vi "AutoLin Protokoll Soll-Ist Abweichung.vi"(10 "Istwerte (ppm)":sgl[](array[numeric]), 11 "Sollwerte (ppm)":sgl[](array[numeric])) -> (1 "% vom Endwert":sgl[](array[numeric]), 2 "% vom Sollwert":sgl[](array[numeric]), 3 "abs. Fehler (ppm)":sgl[](array[numeric]))   [LabVIEW 2020, in "Linearisierung v2.lvlib" / "AutoLin Protokoll.lvlib"]
doc: "Berechnet bei der Kalibrierung die Abweichung der Messdaten des Messgerätes von den Kalibriervorgaben des Gasteilers.\n\nEingangsdaten: 1D-Arrays (SGL) mit N Konzentrationswerten in ppm\n Sollwerte (ppm): Konzentrationswerte Gasteiler\n Istwerte (ppm): Konzentrationswerte Messgerät\n\nAusgangsdaten: Fehler\n abs. Fehler (ppm): Differenz Ist (Messgerät) minus Soll (Gasteiler)\n % vom Sollwert: Differenz bezogen auf Sollwert (Gasteiler)\n % vom Endwert: Differenz bezogen auf Endwert (maximale Konzentration, Gasteiler)"
uses:
  AutoLin Protokoll.lvlib
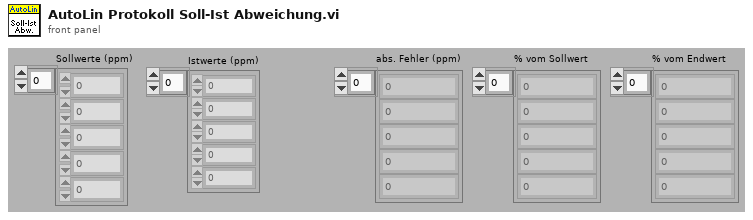
[diagram p1: front panel]
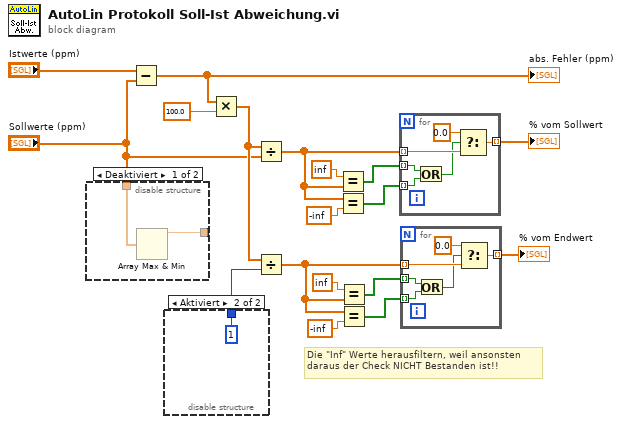
[diagram p0: block diagram]
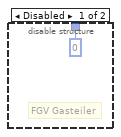
[diagram p2: hidden frame]
diagram:
  # "Die \"Inf\" Werte herausfiltern, weil ansonsten \ndaraus der Check NICHT Bestanden ist!!"
  n1 = disable-structure shown="Deaktiviert" {
    disable-tunnel: [w20 _] -> _
    disable-tunnel: "Sollwerte (ppm)" -> [w19 _]
    frame Disabled {
      n2 = Array Max & Min(array=w19) -> (max value=w20:sgl)  [unwired: 3 out]
    }
    frame Enabled {
    }
  }
  n3 = Subtract(x="Istwerte (ppm)", y="Sollwerte (ppm)") -> (x-y=w16:sgl[])
  "abs. Fehler (ppm)" <- w16
  n4 = disable-structure shown="Aktiviert" {
    disable-tunnel: [u32 0 ("MB-Endwert") u32 1 ("MB-Endwert")] -> w13
    frame Disabled {
      # "FGV Gasteiler"
    }
    frame Enabled {
    }
  }
  n5 = Multiply(x=w16, y=sgl 100.0) -> (x*y=w18:sgl[])
  n6 = Divide(x=w18, y="Sollwerte (ppm)") -> (x/y=w2:sgl[])
  n7 = Divide(x=w18, y=w13) -> (x/y=w9:sgl[])
  n8 = Equal?(x=sgl inf, y=w2) -> (x = y?=w3:bool[])
  n9 = Equal?(x=w2, y=sgl -inf) -> (x = y?=w6:bool[])
  n10 = Equal?(x=sgl inf, y=w9) -> (x = y?=w12:bool[])
  n11 = Equal?(x=w9, y=sgl -inf) -> (x = y?=w7:bool[])
  n12 = for {
    tunnel: w2 -> [w28] mode=indexing
    tunnel: w3 -> [w25] mode=indexing
    tunnel: [w27] -> w1 mode=indexing
    tunnel: w6 -> [w24] mode=indexing
    n13 = Or(x=w25, y=w24) -> (x .or. y?=w23:bool)
    n14 = Select(t=sgl 0.0, s=w23, f=w28) -> (s? t:f=w27:sgl)
  }
  "% vom Sollwert" <- w1
  n15 = for {
    tunnel: w9 -> [w34] mode=indexing
    tunnel: w12 -> [w31] mode=indexing
    tunnel: [w33] -> w10 mode=indexing
    tunnel: w7 -> [w30] mode=indexing
    n16 = Or(x=w31, y=w30) -> (x .or. y?=w29:bool)
    n17 = Select(t=sgl 0.0, s=w29, f=w34) -> (s? t:f=w33:sgl)
  }
  "% vom Endwert" <- w10
